vi "Event Structure 2.vi"() -> ()   [LabVIEW 2020]
panel:
  in  "Stop":bool
  in  "Boolean":bool
  # "Event Structure"
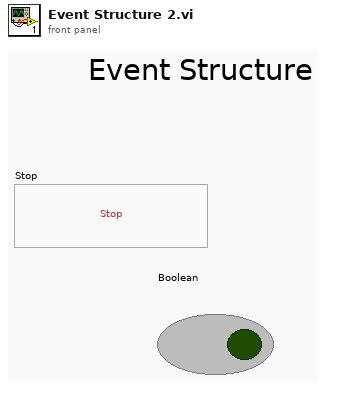
[diagram p1: front panel]
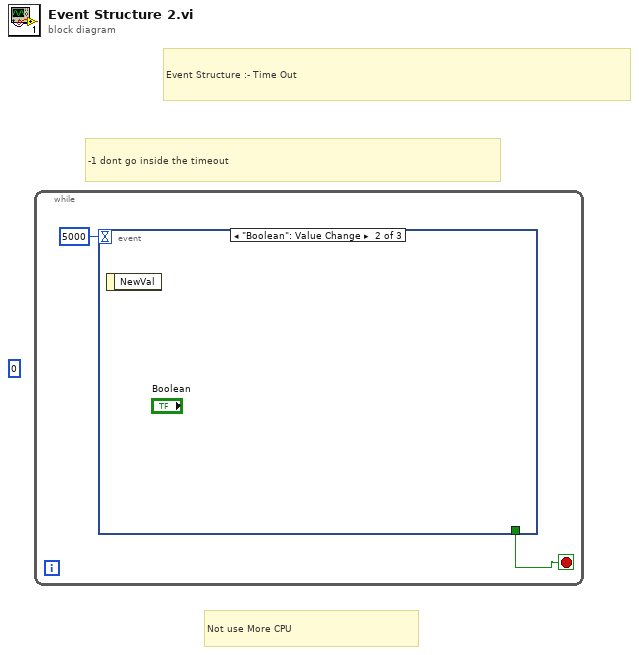
[diagram p0: block diagram]
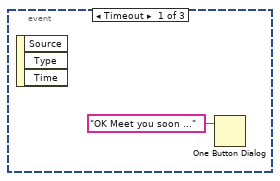
[diagram p2: hidden frame]
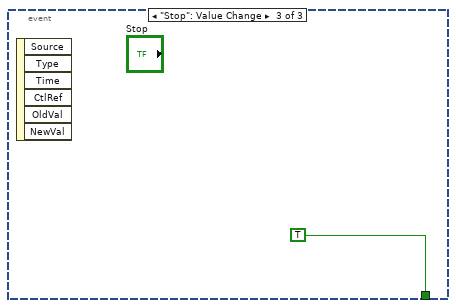
[diagram p3: hidden frame]
diagram:
  (unwired) 0
  # "Not use More CPU"
  # "-1 dont go inside the timeout"
  # "Event Structure :- Time Out"
  n1 = while {
    stop <- w1 stop-if-true
    n2 = event shown="[1] \"Boolean\": Value Change" {
      selector: _ -> [_ _ _]
      dyn-events: _ -> [_ _ _]
      timeout: 5000 -> [_ _ _]
      tunnel: [_ _ TRUE] -> w1
      event Timeout {
        n3 = event-data() -> ()  [unwired: 1 in, 3 out]
        n4 = One Button Dialog(message="OK Meet you soon ...") -> ()  [unwired: 1 in, 1 out]
      }
      event "Boolean": Value Change {
        n5 = event-data() -> ()  [unwired: 1 in, 1 out]
      }
      event "Stop": Value Change {
        n6 = event-data() -> ()  [unwired: 1 in, 6 out]
      }
    }
  }
